vi "configuration UI.vi"() -> ()   [LabVIEW 2013, in "Binary datalogger editor node.lvclass"]
uses:
  Binary datalogger editor node.lvclass
  <vilib>/NI/Tag Bus/tag/tag descriptor.lvclass
  module/configuration/Binary datalogger configuration.lvclass
  <vilib>/NI/Tag Bus Data Framework/Configuration Editor/Classes/Module editor node/module editor node.lvclass
  <vilib>/NI/Module Execution Interface/Engine Configuration/engine configuration.lvclass
  <vilib>/NI/Configuration Framework/Controls/EventCluster.ctl
  <vilib>/NI/Configuration Framework/NISE_CEF_TreeControl.lvlib
  <vilib>/NI/Tag Bus Data Framework/Configuration Editor/Classes/Engine Parent/Engine Parent Editor Node.lvclass
  <vilib>/NI/Configuration Framework/serializable configuration/NISE_CEF_serializable configuration.lvclass
  <vilib>/NI/Tools/Keyed Array/KeyedArray.ctl
  <vilib>/NI/Tools/Keyed Array/Tools_KeyedArray.lvlib
  <vilib>/NI/AMC/Message.ctl
  <vilib>/NI/AMC/AMC.lvlib
  <vilib>/NI/AMC/Message Queue.ctl
  <vilib>/NI/Configuration Framework/Node/NISE_CEF_Node.lvclass
  <vilib>/NI/Configuration Framework/Node/NodeRef.ctl
  <vilib>/NI/Configuration Framework/Node/UserEventRef.ctl
panel:
  in  "Tab Control":T1(tab)
  in  "channels":i32(listbox)
  in  "remove":bool
  in  "avail tags":i32(listbox)=-1
  in  "add all":bool
  in  "add1":bool
  out "Enable Tag":string
  in  "history error":bool
  in  "path error":bool
  in  "Historical Directory":path
  in  "use enable channel":bool
  in  "recalc":bool
  out "Approximate memory usage":dbl
  in  "queue size":u16=2
  in  "scans per write":u16=20
  in  "File Path":path
  in  "user event":T2
  in  "main queue":T3
  in  "node ref":T4
  # "kB"
  # "Note: This value ignores dynamic mapping"
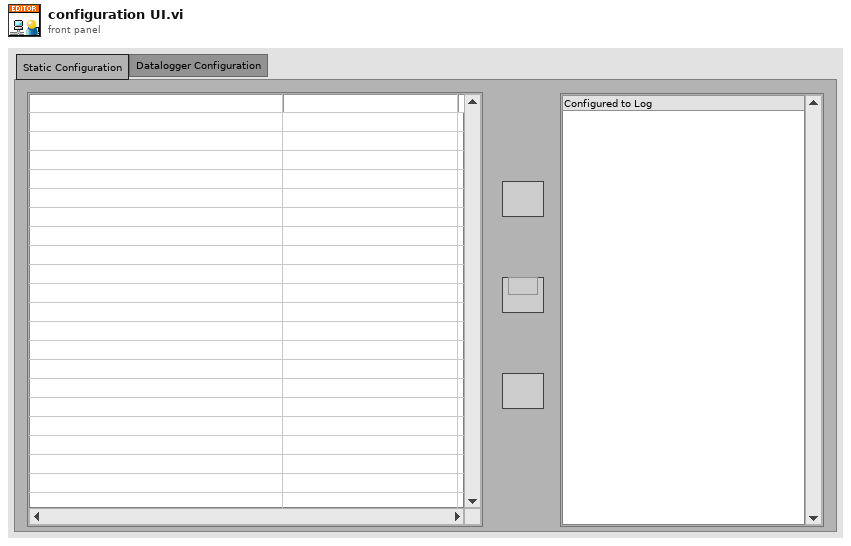
[diagram p1: front panel]
types:
  T1 = enum32{"Static Configuration", "Datalogger Configuration"}
  T2 = typedef "NISE_CEF_Node.lvclass/UserEventRef.ctl" = refnum<user-event>
  T3 = typedef "AMC.lvlib/Message Queue.ctl" = refnum<queue>
  T4 = typedef "NISE_CEF_Node.lvclass/NodeRef.ctl" = refnum<data-value>
  T5 = typedef "NISE_CEF_TreeControl.lvlib/EventCluster.ctl" = cluster{"command":string, "data":string}
  T6 = typedef "tag bus.lvlib/tag descriptor.lvclass/Data Type.ctl" = enum16{"Double", "Single", "I64", "I32", "I16", "I8", "U64", "U32", "U16", "U8", "Boolean", "String", "Array of Double", "Array of Single", "Array of I64", "Array of I32", "Array of I16", "Array of I8", "Array of U64", "Array of U32", "Array of U16", "Array of U8", "Array of Boolean", "Array of String"}
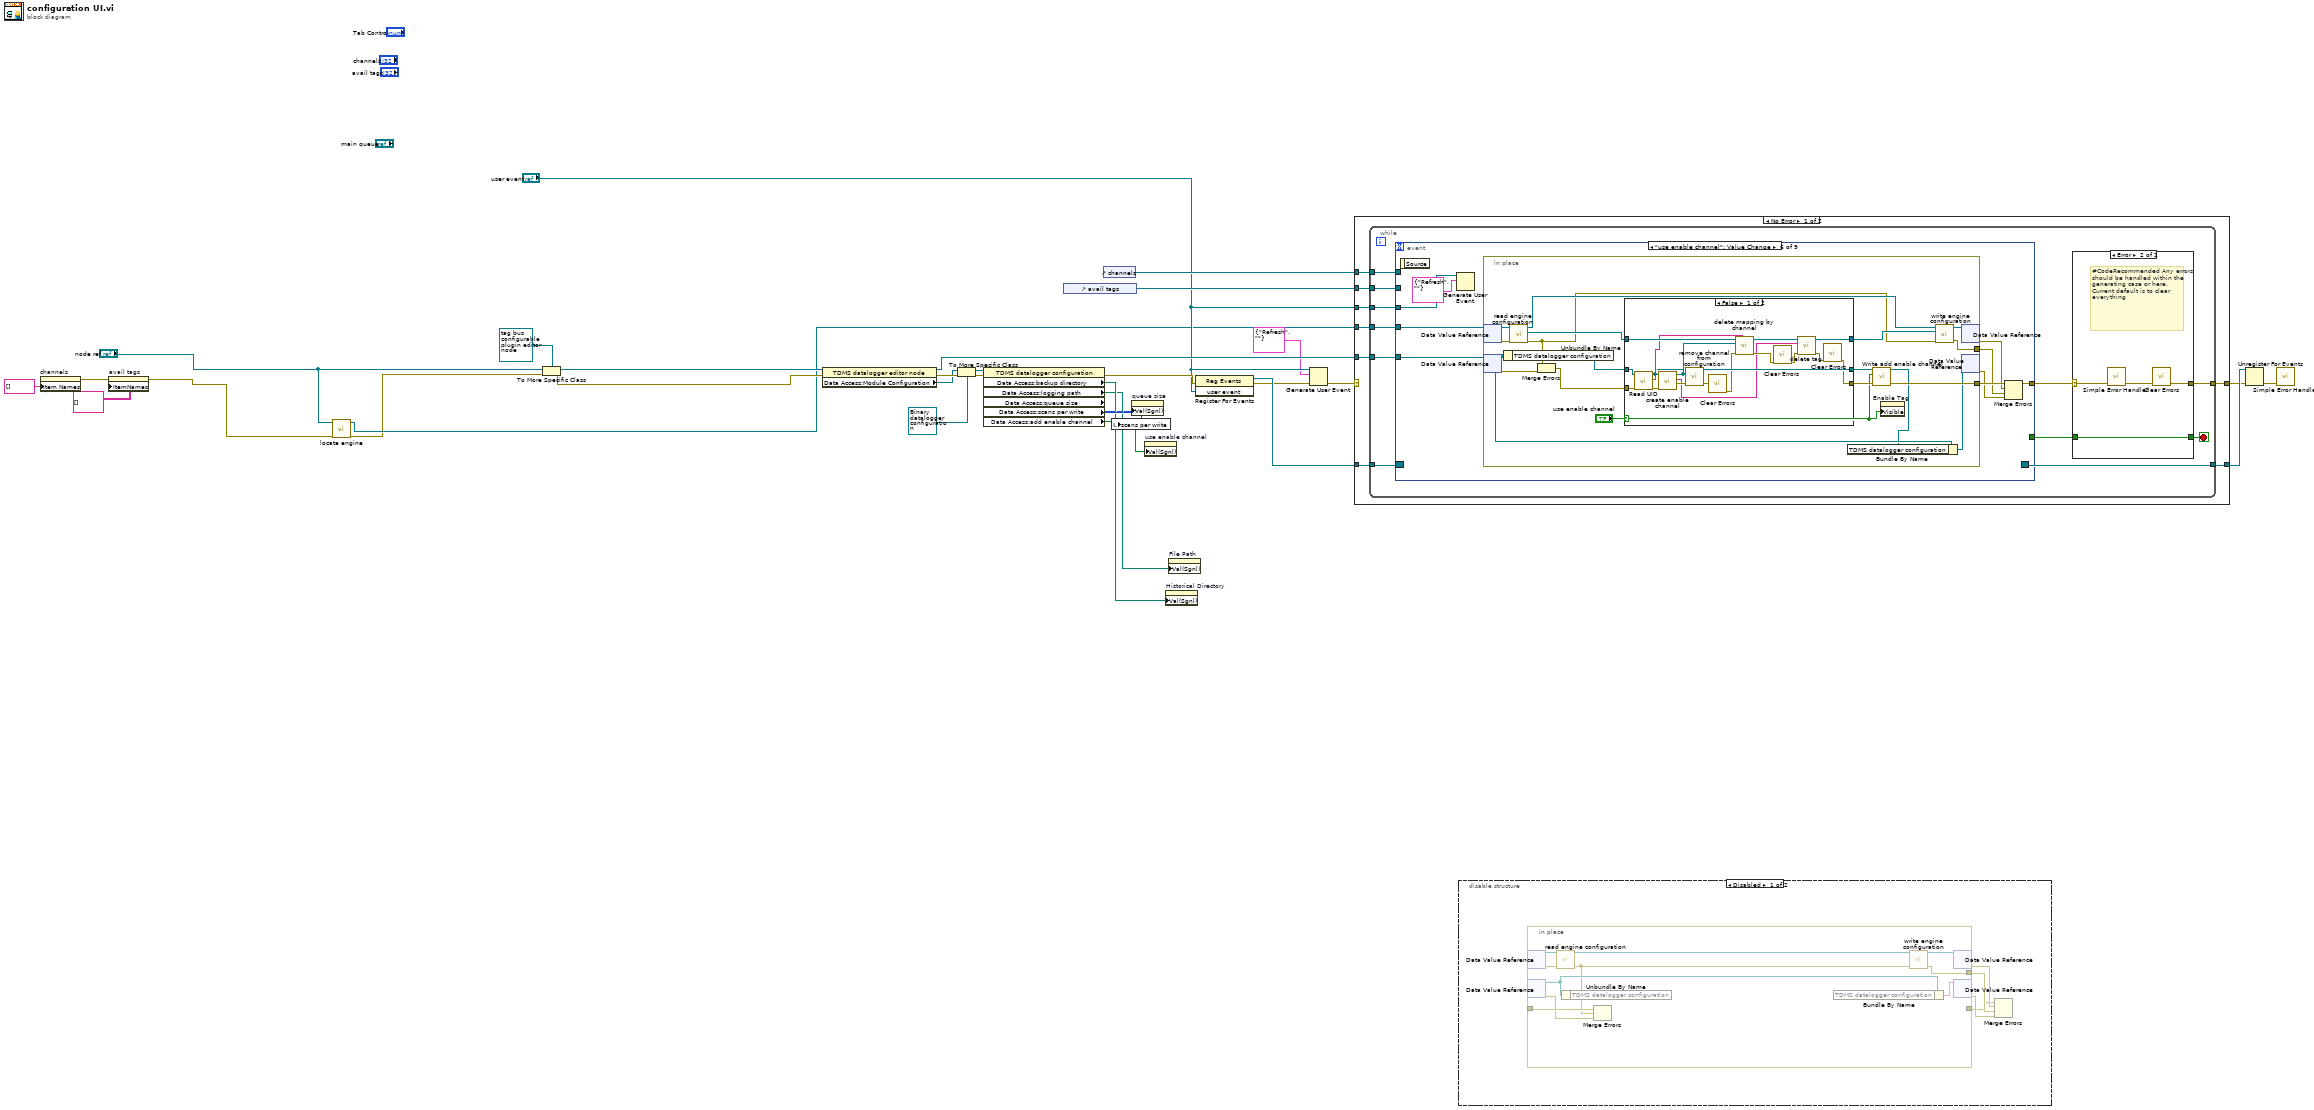
[diagram p0: block diagram]
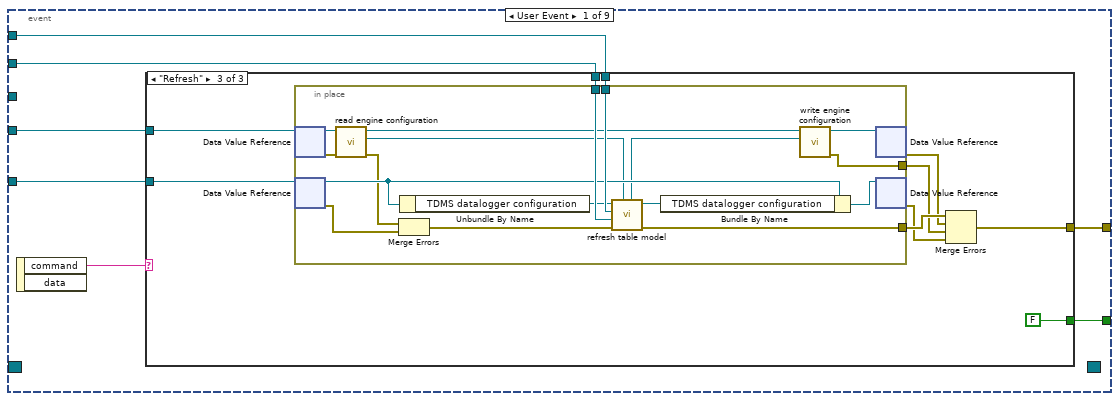
[diagram p3: hidden frame]
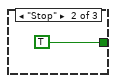
[diagram p5: hidden frame]
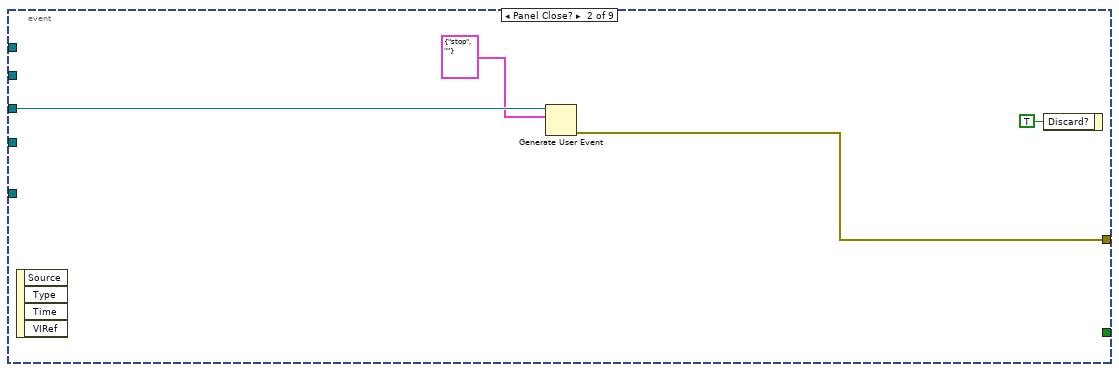
[diagram p6: hidden frame]
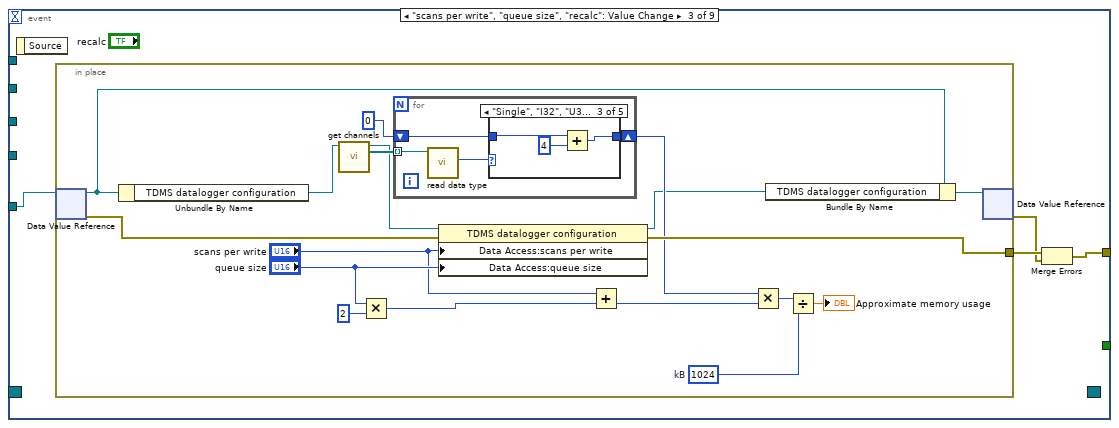
[diagram p7: hidden frame]
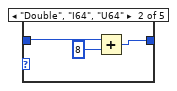
[diagram p9: hidden frame]
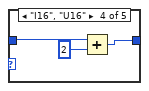
[diagram p10: hidden frame]
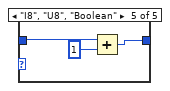
[diagram p11: hidden frame]
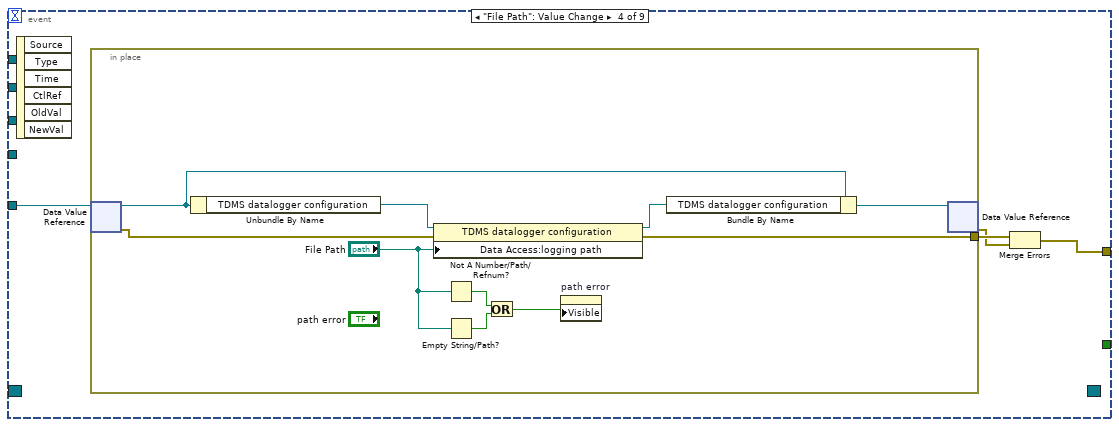
[diagram p12: hidden frame]
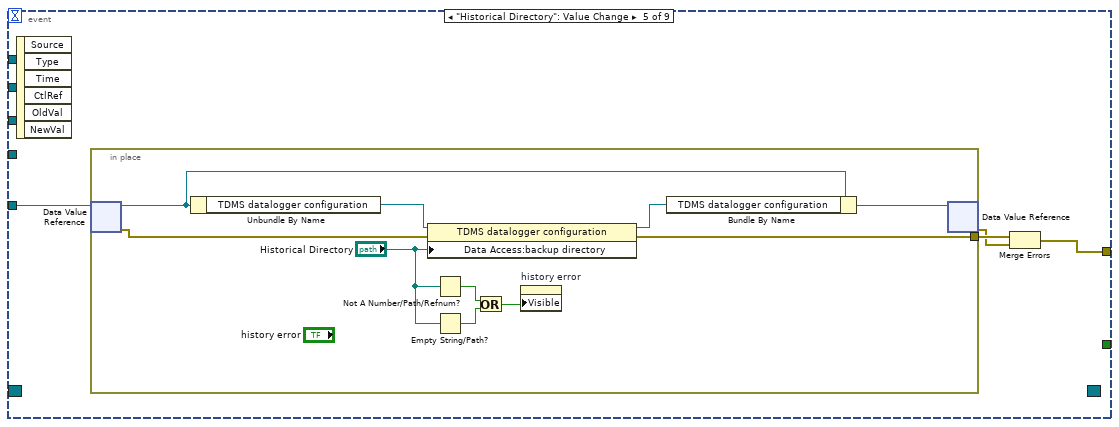
[diagram p13: hidden frame]
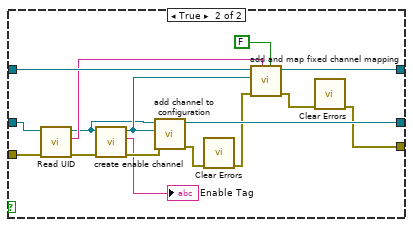
[diagram p14: hidden frame]
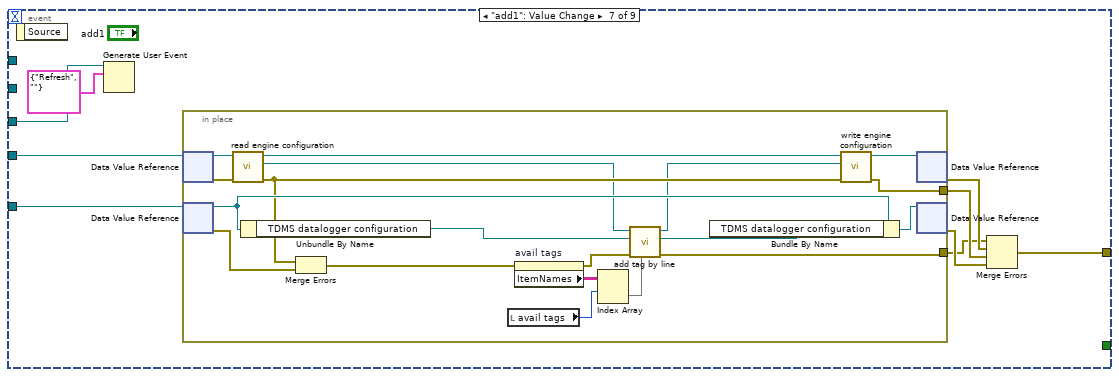
[diagram p15: hidden frame]
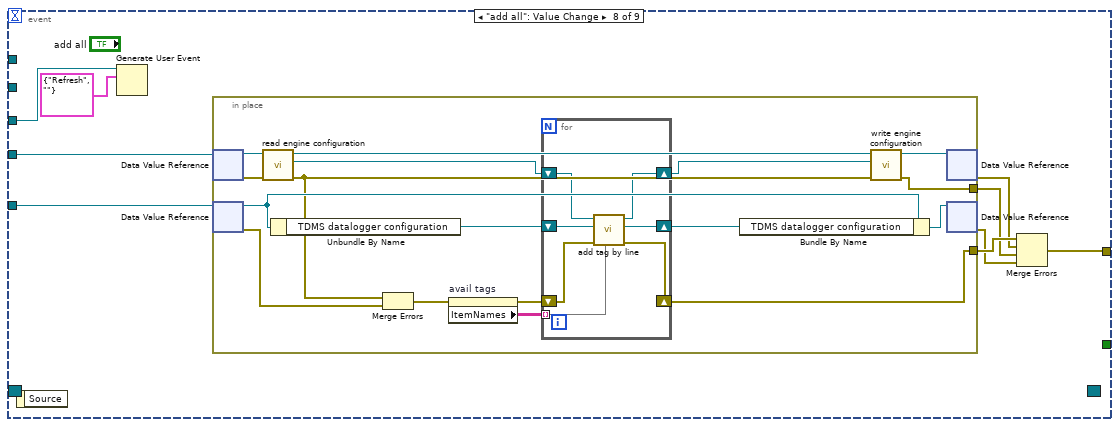
[diagram p16: hidden frame]
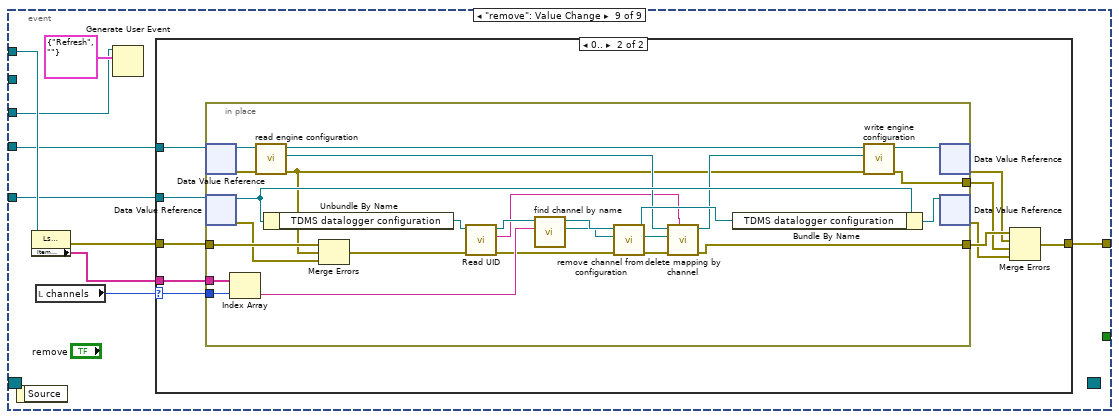
[diagram p17: hidden frame]
diagram:
  n1 = property on="channels" class="LstBox (strict)"("Item Names"=string[] []) -> (error out=w16:errorcluster)  [unwired: 2 in, 1 out]
  n2 = property on="avail tags" class="MCListbox (strict)"(error in=w16, "ItemNames"=string[][] [] ("Item Names")) -> (error out=w7:errorcluster)  [unwired: 1 in, 1 out]
  n3 = call <vilib>:"locate engine.vi"("error in"=w7, "component"="node ref") -> ("error out"=w1:errorcluster, "engine"=w6:refnum<data-value>)  [unwired: 8 in]
  n4 = To More Specific Class(target class=refnum<data-value> refnum ("data value reference"), reference="node ref", error in=w1) -> (specific class reference=w10:refnum<data-value>, error out=w9:errorcluster)
  n5 = property class="TDMS datalogger editor node"(reference=w10, error in=w9) -> (reference out=w12:refnum<data-value>, error out=w29:errorcluster, "Data Access:Module Configuration"=w22:refnum<class "TBM module configuration.lvclass">)
  n6 = To More Specific Class(target class=refnum<class "Binary datalogger configuration.lvclass"> refnum ("bin datalogger configuration"), reference=w22, error in=w29) -> (specific class reference=w20:refnum<class "Binary datalogger configuration.lvclass">, error out=w23:errorcluster)
  n7 = property class="TDMS datalogger configuration"(reference=w20, error in=w23) -> (error out=w19:errorcluster, "Data Access:backup directory"=w26:path, "Data Access:logging path"=w25:path, "Data Access:queue size"=w24:u16, "Data Access:scans per write"=w28:u16, "Data Access:add enable channel"=w27:bool)  [unwired: 1 out]
  n8 = control-ref of="avail tags"() -> (w17:refnum<vi>)
  n9 = control-ref of="channels"() -> (w18:refnum<vi>)
  n10 = local write "scans per write"(w28) -> ()
  n11 = property on="queue size" class="DigNum (strict)"("Val(Sgnl)"=w24) -> ()  [unwired: 2 in, 2 out]
  n12 = property on="use enable channel" class="Bool (strict)"("Val(Sgnl)"=w27) -> ()  [unwired: 2 in, 2 out]
  n13 = property on="Historical Directory" class="Path"("Val(Sgnl)"=w26) -> ()  [unwired: 2 in, 2 out]
  n14 = property on="File Path" class="Path"("Val(Sgnl)"=w25) -> ()  [unwired: 2 in, 2 out]
  n15 = register-events(error in=w19, "user event") -> (reference out=w32:refnum<event-registration>, error out=w4:errorcluster)  [unwired: 1 in]
  n16 = Generate User Event(user event="user event", event data cluster=T5 {"command"="Refresh", "data"=""} ("event data"), error in=w4) -> (error out=w3:errorcluster)  [unwired: 1 in, 1 out]
  n17 = case shown="No Error" w3 {
    selector: w3 -> [_ w332]
    tunnel: w32 -> [w40 w331]
    tunnel: [w39 w331] -> w31
    tunnel: w18 -> [w38 _]
    tunnel: w17 -> [w37 _]
    tunnel: [w36 w332] -> w13
    tunnel: w12 -> [w35 _]
    tunnel: w6 -> [w34 _]
    tunnel: "user event" -> [w33 _]
    frame No Error {
      n18 = while {
        tunnel: w40 -> [w51]
        tunnel: [w50] -> w39
        tunnel: w38 -> [w46]
        tunnel: w37 -> [w45]
        tunnel: w34 -> [w44]
        tunnel: w35 -> [w43]
        tunnel: w33 -> [w42]
        tunnel: [w47] -> w36
        stop <- w48 stop-if-true
        n19 = event shown="[5] \"use enable channel\": Value Change" {
          selector: w51 -> [_ _ _ _ _ _ _ _ _]
          dyn-events: [_ _ _ _ _ _ _ _ _] -> w50
          timeout: _ -> [_ _ _ _ _ _ _ _ _]
          tunnel: [w64 _ _ _ _ _ _ _ _] -> w41
          tunnel: [w62 w95 w98 w138 w152 w169 w225 w255 w294] -> w49
          tunnel: w46 -> [w59 _ _ _ _ _ _ _ w292]
          tunnel: w45 -> [w58 _ _ _ _ _ _ _ _]
          tunnel: w44 -> [w61 _ _ _ _ w167 w226 w253 w286]
          tunnel: w43 -> [w60 _ w99 w137 w151 w168 w227 w254 w287]
          tunnel: w42 -> [_ w94 _ _ _ w171 w232 w260 w288]
          event User Event {
            n20 = event-data() -> ("command"=w63:string)  [unwired: 1 in, 1 out]
            n21 = case shown="\"Refresh\"" w63 {
              tunnel: [_ TRUE FALSE] -> w64
              tunnel: [_ _ w71] -> w62
              tunnel: w61 -> [_ _ w70]
              tunnel: w60 -> [_ _ w69]
              tunnel: w59 -> [_ _ w73]
              tunnel: w58 -> [_ _ w72]
              frame Default {
              }
              frame "Stop" {
              }
              frame "Refresh" {
                n22 = in-place {
                  in-place-border: [w92] -> w74
                  in-place-border: w73 -> [w91]
                  in-place-border: w72 -> [w90]
                  in-place-border: [w76] -> w68
                  n23 = in-place-dvr #1(w70) -> (w80:refnum<class "Engine Parent Editor Node.lvclass">, w81:errorcluster)
                  n24 = in-place-dvr #2(w69) -> (w87:refnum<class "Binary datalogger editor node.lvclass">, w84:errorcluster)
                  n25 = call <vilib>:"read engine configuration.vi"("error in"=w81, "Engine Parent Editor Node in"=w80) -> ("error out"=w77:errorcluster, "engine configuration"=w78:refnum<class "engine configuration.lvclass">, "Engine Parent Editor Node out"=w79:refnum<class "Engine Parent Editor Node.lvclass">)  [unwired: 7 in]
                  n26 = Merge Errors(w77, w84) -> (w89:errorcluster)
                  n27 = Unbundle By Name(w87) -> ("TDMS datalogger configuration"=w88:refnum<class "Binary datalogger configuration.lvclass">)
                  n28 = call "refresh table model.vi"("engine configuration"=w78, "error in"=w89, "avail tags"=w90, "chan table"=w91, "bin datalogger configuration"=w88) -> ("error out"=w92:errorcluster, "bin datalogger configuration out"=w85:refnum<class "Binary datalogger configuration.lvclass">, "engine configuration out"=w82:refnum<class "engine configuration.lvclass">)  [unwired: 4 in]
                  n29 = Bundle By Name(cluster=w87, "TDMS datalogger configuration"=w85) -> (w86:refnum<class "Binary datalogger editor node.lvclass">)
                  n30 = call <vilib>:"write engine configuration.vi"("engine configuration"=w82, "Engine Parent Editor Node in"=w79) -> ("error out"=w76:errorcluster, "Engine Parent Editor Node out"=w83:refnum<class "Engine Parent Editor Node.lvclass">)  [unwired: 8 in]
                  n31 = in-place-dvr #1(w83) -> (w67:errorcluster)  [unwired: 1 out]
                  n32 = in-place-dvr #2(w86) -> (w66:errorcluster)  [unwired: 1 out]
                }
                n33 = Merge Errors(w74, w67, w68, w66) -> (w71:errorcluster)
              }
            }
          }
          event Panel Close? {
            n34 = event-data() -> ()  [unwired: 1 in, 4 out]
            n35 = Generate User Event(user event=w94, event data cluster=T5 {"command"="stop", "data"=""} ("event data")) -> (error out=w95:errorcluster)  [unwired: 2 in, 1 out]
            n36 = event-data("Discard?"=TRUE) -> ()  [unwired: 1 in, 1 out]
          }
          event "scans per write", "queue size", "recalc": Value Change {
            n37 = event-data() -> ()  [unwired: 1 in, 1 out]
            n38 = in-place {
              in-place-border: [w118] -> w100
              w115 = u32 1024  # kB
              n39 = in-place-dvr #3(w99) -> (w108:refnum<class "Binary datalogger editor node.lvclass">, w109:errorcluster)
              n40 = Unbundle By Name(w108) -> ("TDMS datalogger configuration"=w106:refnum<class "Binary datalogger configuration.lvclass">)
              n41 = call-dynamic "get channels.vi"("module configuration in"=w106) -> ("channels"=w112:refnum<class "TBM channel.lvclass">[], "module configuration out"=w110:refnum<class "Binary datalogger configuration.lvclass">)  [unwired: 9 in]
              n42 = Multiply(x="queue size", y=2 ("x")) -> (x*y=w102:i32)
              n43 = for {
                shift-right: [w121] -> w113
                shift-left: u32 0 -> [w122]
                tunnel: w112 -> [w119] mode=indexing
                n44 = call <vilib>:"read data type.vi"("system tag in"=w119) -> ("data type"=w120:T6)  [unwired: 8 in, 2 out]
                n45 = case shown="\"Single\", \"I32\", \"U32\"" w120 {
                  tunnel: w122 -> [w123 w126 w129 w132 w135]
                  tunnel: [w123 w125 w128 w131 w134] -> w121
                  frame Default {
                  }
                  frame "Double", "I64", "U64" {
                    n46 = Add(x=w126, y=u32 8) -> (x+y=w125:u32)
                  }
                  frame "Single", "I32", "U32" {
                    n47 = Add(x=w129, y=u32 4) -> (x+y=w128:u32)
                  }
                  frame "I16", "U16" {
                    n48 = Add(x=w132, y=u32 2) -> (x+y=w131:u32)
                  }
                  frame "I8", "U8", "Boolean" {
                    n49 = Add(x=w135, y=u32 1) -> (x+y=w134:u32)
                  }
                }
              }
              n50 = property class="TDMS datalogger configuration"(reference=w110, error in=w109, "Data Access:scans per write"="scans per write", "Data Access:queue size"="queue size") -> (reference out=w105:refnum<class "Binary datalogger configuration.lvclass">, error out=w118:errorcluster)
              n51 = Add(x="scans per write", y=w102) -> (x+y=w103:i32)
              n52 = Multiply(x=w113, y=w103) -> (x*y=w104:u32)
              n53 = Bundle By Name(cluster=w108, "TDMS datalogger configuration"=w105) -> (w107:refnum<class "Binary datalogger editor node.lvclass">)
              n54 = Divide(x=w104, y=w115) -> (x/y=→"Approximate memory usage":dbl)
              n55 = in-place-dvr #3(w107) -> (w97:errorcluster)  [unwired: 1 out]
            }
            n56 = Merge Errors(w100, w97) -> (w98:errorcluster)
          }
          event "File Path": Value Change {
            n57 = event-data() -> ()  [unwired: 1 in, 6 out]
            n58 = in-place {
              in-place-border: [w149] -> w139
              n59 = in-place-dvr #4(w137) -> (w140:refnum<class "Binary datalogger editor node.lvclass">, w143:errorcluster)
              n60 = Unbundle By Name(w140) -> ("TDMS datalogger configuration"=w144:refnum<class "Binary datalogger configuration.lvclass">)
              n61 = property class="TDMS datalogger configuration"(reference=w144, error in=w143, "Data Access:logging path"="File Path") -> (reference out=w142:refnum<class "Binary datalogger configuration.lvclass">, error out=w149:errorcluster)
              n62 = Not A Number/Path/Refnum?(number/path/refnum="File Path") -> (NaN/Path/Refnum?=w146:bool)
              n63 = Empty String/Path?(string/path="File Path") -> (empty?=w147:bool)
              n64 = Or(x=w146, y=w147) -> (x .or. y?=w145:bool)
              n65 = property on="path error" class="Bool"("Visible"=w145) -> ()  [unwired: 2 in, 2 out]
              n66 = Bundle By Name(cluster=w140, "TDMS datalogger configuration"=w142) -> (w141:refnum<class "Binary datalogger editor node.lvclass">)
              n67 = in-place-dvr #4(w141) -> (w136:errorcluster)  [unwired: 1 out]
            }
            n68 = Merge Errors(w139, w136) -> (w138:errorcluster)
          }
          event "Historical Directory": Value Change {
            n69 = event-data() -> ()  [unwired: 1 in, 6 out]
            n70 = in-place {
              in-place-border: [w157] -> w153
              n71 = in-place-dvr #5(w151) -> (w162:refnum<class "Binary datalogger editor node.lvclass">, w154:errorcluster)
              n72 = Unbundle By Name(w162) -> ("TDMS datalogger configuration"=w155:refnum<class "Binary datalogger configuration.lvclass">)
              n73 = property class="TDMS datalogger configuration"(reference=w155, error in=w154, "Data Access:backup directory"="Historical Directory") -> (reference out=w156:refnum<class "Binary datalogger configuration.lvclass">, error out=w157:errorcluster)
              n74 = Not A Number/Path/Refnum?(number/path/refnum="Historical Directory") -> (NaN/Path/Refnum?=w160:bool)
              n75 = Empty String/Path?(string/path="Historical Directory") -> (empty?=w161:bool)
              n76 = Or(x=w160, y=w161) -> (x .or. y?=w158:bool)
              n77 = property on="history error" class="Bool"("Visible"=w158) -> ()  [unwired: 2 in, 2 out]
              n78 = Bundle By Name(cluster=w162, "TDMS datalogger configuration"=w156) -> (w163:refnum<class "Binary datalogger editor node.lvclass">)
              n79 = in-place-dvr #5(w163) -> (w150:errorcluster)  [unwired: 1 out]
            }
            n80 = Merge Errors(w153, w150) -> (w152:errorcluster)
          }
          event "use enable channel": Value Change {
            n81 = event-data() -> ()  [unwired: 1 in, 1 out]
            n82 = Generate User Event(user event=w171, event data cluster=T5 {"command"="Refresh", "data"=""} ("event data")) -> ()  [unwired: 2 in, 2 out]
            n83 = in-place {
              in-place-border: [w188] -> w170
              in-place-border: [w182] -> w165
              n84 = in-place-dvr #6(w167) -> (w186:refnum<class "Engine Parent Editor Node.lvclass">, w184:errorcluster)
              n85 = in-place-dvr #7(w168) -> (w180:refnum<class "Binary datalogger editor node.lvclass">, w183:errorcluster)
              n86 = Unbundle By Name(w180) -> ("TDMS datalogger configuration"=w181:refnum<class "Binary datalogger configuration.lvclass">)
              n87 = call <vilib>:"read engine configuration.vi"("error in"=w184, "Engine Parent Editor Node in"=w186) -> ("error out"=w174:errorcluster, "engine configuration"=w185:refnum<class "engine configuration.lvclass">, "Engine Parent Editor Node out"=w176:refnum<class "Engine Parent Editor Node.lvclass">)  [unwired: 7 in]
              n88 = Merge Errors(w174, w183) -> (w173:errorcluster)
              n89 = case shown="False" "use enable channel" {
                tunnel: [w203 w224] -> w175
                tunnel: w185 -> [w206 w220]
                tunnel: [w208 w223] -> w190
                tunnel: w181 -> [w194 w213]
                tunnel: [w199 w218] -> w189
                tunnel: w173 -> [w196 w215]
                frame False {
                  n90 = call <vilib>:"Read UID.vi"("error in"=w196, "configuration in"=w194) -> ("error out"=w195:errorcluster, "instance id"=w193:string, "configuration out"=w192:refnum<class "Binary datalogger configuration.lvclass">)  [unwired: 7 in]
                  n91 = call "create enable channel.vi"("error in"=w195, "bin datalogger configuration"=w192) -> ("error out"=w207:errorcluster, "enable channel name"=w191:string, "enable channel"=w205:refnum<class "TBM channel.lvclass">)  [unwired: 7 in]
                  n92 = call "remove channel from configuration.vi"("error in"=w207, "TBM channel in"=w205, "bin datalogger configuration in"=w192) -> ("error out"=w198:errorcluster, "bin datalogger configuration out"=w208:refnum<class "Binary datalogger configuration.lvclass">)  [unwired: 7 in]
                  n93 = call <vilib>:"Clear Errors.vi"("error in (no error)"=w198) -> ("error out"=w197:errorcluster)  [unwired: 6 in]
                  n94 = call <vilib>:"delete mapping by channel.vi"("owner ID"=w193, "error in"=w197, "channel"=w205, "engine configuration in"=w206) -> ("error out"=w201:errorcluster, "engine configuration out"=w204:refnum<class "engine configuration.lvclass">)  [unwired: 6 in]
                  n95 = call <vilib>:"Clear Errors.vi"("error in (no error)"=w201) -> ("error out"=w202:errorcluster)  [unwired: 6 in]
                  n96 = call <vilib>:"delete tag.vi"("error in"=w202, "tag name"=w191, "engine configuration in"=w204) -> ("error out"=w200:errorcluster, "engine configuration out"=w203:refnum<class "engine configuration.lvclass">)  [unwired: 7 in]
                  n97 = call <vilib>:"Clear Errors.vi"("error in (no error)"=w200) -> ("error out"=w199:errorcluster)  [unwired: 6 in]
                }
                frame True {
                  n98 = call <vilib>:"Read UID.vi"("error in"=w215, "configuration in"=w213) -> ("error out"=w214:errorcluster, "instance id"=w212:string, "configuration out"=w210:refnum<class "Binary datalogger configuration.lvclass">)  [unwired: 7 in]
                  n99 = call "create enable channel.vi"("error in"=w214, "bin datalogger configuration"=w210) -> ("error out"=w222:errorcluster, "enable channel name"=→"Enable Tag":string, "enable channel"=w221:refnum<class "TBM channel.lvclass">)  [unwired: 7 in]
                  n100 = call "add channel to configuration.vi"("error in"=w222, "TBM channel in"=w221, "bin datalogger configuration in"=w210) -> ("error out"=w217:errorcluster, "bin datalogger configuration out"=w223:refnum<class "Binary datalogger configuration.lvclass">)  [unwired: 7 in]
                  n101 = call <vilib>:"Clear Errors.vi"("error in (no error)"=w217) -> ("error out"=w216:errorcluster)  [unwired: 6 in]
                  n102 = call <vilib>:"add and map fixed channel mapping.vi"("set module as owner"=FALSE, "module instance"=w212, "error in"=w216, "fixed channel"=w221, "engine configuration in"=w220) -> ("error out"=w219:errorcluster, "engine configuration out"=w224:refnum<class "engine configuration.lvclass">)  [unwired: 5 in]
                  n103 = call <vilib>:"Clear Errors.vi"("error in (no error)"=w219) -> ("error out"=w218:errorcluster)  [unwired: 6 in]
                }
              }
              n104 = call "Write add enable channel.vi"("error in (no error)"=w189, "add enable channel"="use enable channel", "bin datalogger configuration in"=w190) -> ("error out"=w188:errorcluster, "bin datalogger configuration out"=w179:refnum<class "Binary datalogger configuration.lvclass">)  [unwired: 7 in]
              n105 = Bundle By Name(cluster=w180, "TDMS datalogger configuration"=w179) -> (w178:refnum<class "Binary datalogger editor node.lvclass">)
              n106 = property on="Enable Tag" class="Str"("Visible"="use enable channel") -> ()  [unwired: 2 in, 2 out]
              n107 = call <vilib>:"write engine configuration.vi"("error in"=w174, "engine configuration"=w175, "Engine Parent Editor Node in"=w176) -> ("error out"=w182:errorcluster, "Engine Parent Editor Node out"=w177:refnum<class "Engine Parent Editor Node.lvclass">)  [unwired: 7 in]
              n108 = in-place-dvr #6(w177) -> (w166:errorcluster)  [unwired: 1 out]
              n109 = in-place-dvr #7(w178) -> (w164:errorcluster)  [unwired: 1 out]
            }
            n110 = Merge Errors(w170, w166, w165, w164) -> (w169:errorcluster)
          }
          event "add1": Value Change {
            n111 = event-data() -> ()  [unwired: 1 in, 1 out]
            n112 = Generate User Event(user event=w232, event data cluster=T5 {"command"="Refresh", "data"=""} ("event data")) -> ()  [unwired: 2 in, 2 out]
            n113 = in-place {
              in-place-border: [w237] -> w228
              in-place-border: [w246] -> w229
              n114 = in-place-dvr #8(w226) -> (w248:refnum<class "Engine Parent Editor Node.lvclass">, w249:errorcluster)
              n115 = in-place-dvr #9(w227) -> (w245:refnum<class "Binary datalogger editor node.lvclass">, w251:errorcluster)
              n116 = call <vilib>:"read engine configuration.vi"("error in"=w249, "Engine Parent Editor Node in"=w248) -> ("error out"=w244:errorcluster, "engine configuration"=w235:refnum<class "engine configuration.lvclass">, "Engine Parent Editor Node out"=w247:refnum<class "Engine Parent Editor Node.lvclass">)  [unwired: 7 in]
              n117 = Unbundle By Name(w245) -> ("TDMS datalogger configuration"=w239:refnum<class "Binary datalogger configuration.lvclass">)
              n118 = Merge Errors(w244, w251) -> (w234:errorcluster)
              n119 = local read "avail tags"() -> (w241:i32)
              n120 = property on="avail tags" class="MCListbox (strict)"(error in=w234) -> (error out=w242:errorcluster, "ItemNames"=w240:string[][])  [unwired: 1 in, 1 out]
              n121 = Index Array(array=w240, index (row)=w241) -> (element=w243:string[])  [unwired: 1 in]
              n122 = call "add tag by line.vi"("ItemNames"=w243, "error in"=w242, "bin datalogger configuration in"=w239, "engine configuration in"=w235) -> ("error out"=w237:errorcluster, "bin datalogger configuration out"=w238:refnum<class "Binary datalogger configuration.lvclass">, "engine configuration out"=w236:refnum<class "engine configuration.lvclass">)  [unwired: 5 in]
              n123 = Bundle By Name(cluster=w245, "TDMS datalogger configuration"=w238) -> (w252:refnum<class "Binary datalogger editor node.lvclass">)
              n124 = call <vilib>:"write engine configuration.vi"("error in"=w244, "engine configuration"=w236, "Engine Parent Editor Node in"=w247) -> ("error out"=w246:errorcluster, "Engine Parent Editor Node out"=w250:refnum<class "Engine Parent Editor Node.lvclass">)  [unwired: 7 in]
              n125 = in-place-dvr #8(w250) -> (w230:errorcluster)  [unwired: 1 out]
              n126 = in-place-dvr #9(w252) -> (w231:errorcluster)  [unwired: 1 out]
            }
            n127 = Merge Errors(w228, w230, w229, w231) -> (w225:errorcluster)
          }
          event "add all": Value Change {
            n128 = event-data() -> ()  [unwired: 1 in, 1 out]
            n129 = Generate User Event(user event=w260, event data cluster=T5 {"command"="Refresh", "data"=""} ("event data")) -> ()  [unwired: 2 in, 2 out]
            n130 = in-place {
              in-place-border: [w263] -> w259
              in-place-border: [w272] -> w258
              n131 = in-place-dvr #10(w253) -> (w274:refnum<class "Engine Parent Editor Node.lvclass">, w275:errorcluster)
              n132 = in-place-dvr #11(w254) -> (w271:refnum<class "Binary datalogger editor node.lvclass">, w277:errorcluster)
              n133 = call <vilib>:"read engine configuration.vi"("error in"=w275, "Engine Parent Editor Node in"=w274) -> ("error out"=w270:errorcluster, "engine configuration"=w265:refnum<class "engine configuration.lvclass">, "Engine Parent Editor Node out"=w273:refnum<class "Engine Parent Editor Node.lvclass">)  [unwired: 7 in]
              n134 = Unbundle By Name(w271) -> ("TDMS datalogger configuration"=w266:refnum<class "Binary datalogger configuration.lvclass">)
              n135 = Merge Errors(w270, w277) -> (w262:errorcluster)
              n136 = property on="avail tags" class="MCListbox (strict)"(error in=w262) -> (error out=w268:errorcluster, "ItemNames"=w269:string[][])  [unwired: 1 in, 1 out]
              n137 = for {
                tunnel: w269 -> [w279] mode=indexing
                shift-right: [w284] -> w263
                shift-left: w268 -> [w282]
                shift-right: [w285] -> w267
                shift-left: w266 -> [w283]
                shift-right: [w280] -> w264
                shift-left: w265 -> [w281]
                n138 = call "add tag by line.vi"("ItemNames"=w279, "error in"=w282, "bin datalogger configuration in"=w283, "engine configuration in"=w281) -> ("error out"=w284:errorcluster, "bin datalogger configuration out"=w285:refnum<class "Binary datalogger configuration.lvclass">, "engine configuration out"=w280:refnum<class "engine configuration.lvclass">)  [unwired: 5 in]
              }
              n139 = Bundle By Name(cluster=w271, "TDMS datalogger configuration"=w267) -> (w278:refnum<class "Binary datalogger editor node.lvclass">)
              n140 = call <vilib>:"write engine configuration.vi"("error in"=w270, "engine configuration"=w264, "Engine Parent Editor Node in"=w273) -> ("error out"=w272:errorcluster, "Engine Parent Editor Node out"=w276:refnum<class "Engine Parent Editor Node.lvclass">)  [unwired: 7 in]
              n141 = in-place-dvr #10(w276) -> (w257:errorcluster)  [unwired: 1 out]
              n142 = in-place-dvr #11(w278) -> (w256:errorcluster)  [unwired: 1 out]
            }
            n143 = Merge Errors(w259, w257, w258, w256) -> (w255:errorcluster)
          }
          event "remove": Value Change {
            n144 = event-data() -> ()  [unwired: 1 in, 1 out]
            n145 = property class="LstBox (strict)"(reference=w292) -> (error out=w291:errorcluster, "Item Names"=w293:string[])  [unwired: 1 in, 1 out]
            n146 = local read "channels"() -> (w290:i32)
            n147 = Generate User Event(user event=w288, event data cluster=T5 {"command"="Refresh", "data"=""} ("event data")) -> ()  [unwired: 2 in, 2 out]
            n148 = case shown="0.." w290 {
              selector: w290 -> [_ w296]
              tunnel: [w295 w301] -> w294
              tunnel: w293 -> [_ w297]
              tunnel: w291 -> [w295 w298]
              tunnel: w287 -> [_ w300]
              tunnel: w286 -> [_ w299]
              frame ..-1 {
              }
              frame 0.. {
                n149 = in-place {
                  in-place-border: w298 -> [w330]
                  in-place-border: [w312] -> w305
                  in-place-border: [w323] -> w304
                  in-place-border: w297 -> [w315]
                  in-place-border: w296 -> [w314]
                  n150 = in-place-dvr #12(w299) -> (w325:refnum<class "Engine Parent Editor Node.lvclass">, w326:errorcluster)
                  n151 = in-place-dvr #13(w300) -> (w322:refnum<class "Binary datalogger editor node.lvclass">, w328:errorcluster)
                  n152 = Index Array(array=w315, index=w314) -> (element=w319:string)
                  n153 = call <vilib>:"read engine configuration.vi"("error in"=w326, "Engine Parent Editor Node in"=w325) -> ("error out"=w310:errorcluster, "engine configuration"=w313:refnum<class "engine configuration.lvclass">, "Engine Parent Editor Node out"=w324:refnum<class "Engine Parent Editor Node.lvclass">)  [unwired: 7 in]
                  n154 = Unbundle By Name(w322) -> ("TDMS datalogger configuration"=w308:refnum<class "Binary datalogger configuration.lvclass">)
                  n155 = Merge Errors(w330, w310, w328) -> (w316:errorcluster)
                  n156 = call <vilib>:"Read UID.vi"("error in"=w316, "configuration in"=w308) -> ("error out"=w309:errorcluster, "instance id"=w306:string, "configuration out"=w307:refnum<class "Binary datalogger configuration.lvclass">)  [unwired: 7 in]
                  n157 = call "find channel by name.vi"("channel name"=w319, "bin datalogger configuration in"=w307) -> ("channel"=w318:refnum<class "TBM channel.lvclass">, "bin datalogger configuration out"=w320:refnum<class "Binary datalogger configuration.lvclass">)  [unwired: 8 in]
                  n158 = call "remove channel from configuration.vi"("error in"=w309, "TBM channel in"=w318, "bin datalogger configuration in"=w320) -> ("error out"=w321:errorcluster, "bin datalogger configuration out"=w317:refnum<class "Binary datalogger configuration.lvclass">)  [unwired: 7 in]
                  n159 = call <vilib>:"delete mapping by channel.vi"("owner ID"=w306, "error in"=w321, "channel"=w318, "engine configuration in"=w313) -> ("error out"=w312:errorcluster, "engine configuration out"=w311:refnum<class "engine configuration.lvclass">)  [unwired: 6 in]
                  n160 = Bundle By Name(cluster=w322, "TDMS datalogger configuration"=w317) -> (w329:refnum<class "Binary datalogger editor node.lvclass">)
                  n161 = call <vilib>:"write engine configuration.vi"("error in"=w310, "engine configuration"=w311, "Engine Parent Editor Node in"=w324) -> ("error out"=w323:errorcluster, "Engine Parent Editor Node out"=w327:refnum<class "Engine Parent Editor Node.lvclass">)  [unwired: 7 in]
                  n162 = in-place-dvr #12(w327) -> (w303:errorcluster)  [unwired: 1 out]
                  n163 = in-place-dvr #13(w329) -> (w302:errorcluster)  [unwired: 1 out]
                }
                n164 = Merge Errors(w305, w303, w304, w302) -> (w301:errorcluster)
              }
            }
          }
        }
        n165 = case shown="Error" w49 {
          selector: w49 -> [w52 w56]
          tunnel: [w53 w57] -> w48
          tunnel: w41 -> [w53 w57]
          tunnel: [w52 w54] -> w47
          frame No Error {
          }
          frame Error {
            # "#CodeRecommended Any errors should be handled within the generating case or here. Current default is to clear everything"
            n166 = call <vilib>:"Simple Error Handler.vi"("error in (no error)"=w56) -> ("error out"=w55:errorcluster)  [unwired: 4 in, 4 out]
            n167 = call <vilib>:"Clear Errors.vi"("error in (no error)"=w55) -> ("error out"=w54:errorcluster)  [unwired: 6 in]
          }
        }
      }
    }
    frame Error {
    }
  }
  n168 = disable-structure shown="Disabled" {
    frame Disabled {
      n169 = in-place {
        in-place-border: _ -> [w346]
        in-place-border: [_] -> w333
        in-place-border: [w339] -> w334
        n170 = in-place-dvr #14() -> (w341:refnum<class "Engine Parent Editor Node.lvclass">, w342:errorcluster)  [unwired: 1 in]
        n171 = in-place-dvr #15() -> (w338:refnum<class "TDMS datalogger editor node.lvclass">, w344:errorcluster)  [unwired: 1 in]
        n172 = call <vilib>:"read engine configuration.vi"("error in"=w342, "Engine Parent Editor Node in"=w341) -> ("error out"=w337:errorcluster, "Engine Parent Editor Node out"=w340:refnum<class "Engine Parent Editor Node.lvclass">)  [unwired: 7 in, 1 out]
        n173 = Unbundle By Name(w338) -> ()  [unwired: 1 out]
        n174 = Merge Errors(w346, w337, w344) -> ()  [unwired: 1 out]
        n175 = Bundle By Name(cluster=w338) -> (w345:cluster{})  [unwired: 1 in]
        n176 = call <vilib>:"write engine configuration.vi"("error in"=w337, "Engine Parent Editor Node in"=w340) -> ("error out"=w339:errorcluster, "Engine Parent Editor Node out"=w343:refnum<class "Engine Parent Editor Node.lvclass">)  [unwired: 8 in]
        n177 = in-place-dvr #14(w343) -> (w335:errorcluster)  [unwired: 1 out]
        n178 = in-place-dvr #15(w345) -> (w336:errorcluster)  [unwired: 1 out]
      }
      n179 = Merge Errors(w333, w335, w334, w336) -> ()  [unwired: 1 out]
    }
    frame Enabled {
    }
  }
  n180 = Unregister For Events(event registration refnum=w31, error in=w13) -> (error out=w30:errorcluster)
  n181 = call <vilib>:"Simple Error Handler.vi"("error in (no error)"=w30) -> ()  [unwired: 4 in, 5 out]
